vi "MultiplexerSerialInterfaceHost.vi"() -> ()   [LabVIEW 2016]
uses:
  <vilib>/FPGAPlugInAG/USB-7856R OEM/niLvFpga_Open_USB-7856R OEM.vi
  <vilib>/rvi/interface/common/dynamic/niFpgaDynamicAddResources.vi
  <vilib>/Utility/error.llb/Error Cluster From Error Code.vi
  <vilib>/rvi/errors/niLvFpgaAdjustHostInterfaceError.vi
  <vilib>/FPGAPlugInAG/Dynamic/niLvFpga_Close_Dynamic.vi
  <vilib>/rvi/interface/nirviOpenFPGA/nirviOpenFPGA.xnode
  FPGA Bitfiles/qnmController797_usbRIO_MultiplexerSPIFPGA.lvbitx
  <vilib>/rvi/interface/nirviReadWriteControl/nirviReadWriteControl.xnode
  <vilib>/rvi/interface/nirviCloseFPGA/nirviCloseFPGA.xnode
  NiFpgaLv.dll
  <vilib>/rvi/interface/Simulation/niFpgaSimulationCallBeginRW.vi
panel:
  in  "Buffer":T1={"Update Multiplexer"=FALSE, "Channel #"=0, "Dimension"=32, "Selection"=0, "Clock delay"=50} {"Selection" items=["AO0 (X)", "AO1 (Y)", "AO2 (Z)", "AO3 (DRIVE)", "AO4 (BIAS)", "AO5 (STICK-SLIP X - DC Motor)", "AO6 (STICK-SLIP Y)", "AO7 (STICK-SLIP Z )", "AI0 (Deflection)", "AI1 (Horizontal)", "AI2 (Sum)", "AI3", "AI4", "AI5", "AI6", "AI7"]; "Channel #" max=32}
  in  "Output Enable":bool
  in  "VGA":T2={"Update"=FALSE, "Dimension"=32, "Selection"=0, "Clock delay"=50, "Gain (dB)"=0} {"Gain (dB)" max=40; "Selection" items=["AO0 (X)", "AO1 (Y)", "AO2 (Z)", "AO3 (DRIVE)", "AO4 (BIAS)", "AO5 (STICK-SLIP X - DC Motor)", "AO6 (STICK-SLIP Y)", "AO7 (STICK-SLIP Z )", "AI0 (Deflection)", "AI1 (Horizontal)", "AI2 (Sum)", "AI3", "AI4", "AI5", "AI6", "AI7"]}
  in  "Multiplexer":T1={"Update Multiplexer"=FALSE, "Channel #"=0, "Dimension"=32, "Selection"=0, "Clock delay"=50} {"Selection" items=["AO0 (X)", "AO1 (Y)", "AO2 (Z)", "AO3 (DRIVE)", "AO4 (BIAS)", "AO5 (STICK-SLIP X - DC Motor)", "AO6 (STICK-SLIP Y)", "AO7 (STICK-SLIP Z )", "AI0 (Deflection)", "AI1 (Horizontal)", "AI2 (Sum)", "AI3", "AI4", "AI5", "AI6", "AI7"]; "Channel #" max=32}
  in  "Frequency":u16(ring) items=["AO0 (X)", "AO1 (Y)", "AO2 (Z)", "AO3 (DRIVE)", "AO4 (BIAS)", "AO5 (STICK-SLIP X - DC Motor)", "AO6 (STICK-SLIP Y)", "AO7 (STICK-SLIP Z )", "AI0 (Deflection)", "AI1 (Horizontal)", "AI2 (Sum)", "AI3", "AI4", "AI5", "AI6", "AI7"]
  in  "Clock delay 2":u32=50
  in  "Dimension 2":u8=32
  in  "Line #":u8 max=32
  in  "Update Quad Multiplier":bool
  # "Buffer"
  # "VGA"
  # "HMC960LP4E"
  # "DAC8554"
  # "Quad Multiplier"
  # "Multiplexer"
  # "HV5122"
  # "DAC8803"
  # "Select the element"
  # "Select the element"
  # "Select the element"
  # "Select the element"
  # "MICROCHIP"
  # "TEXAS INSTRUMENTS"
  # "Serial to Parallel Converter"
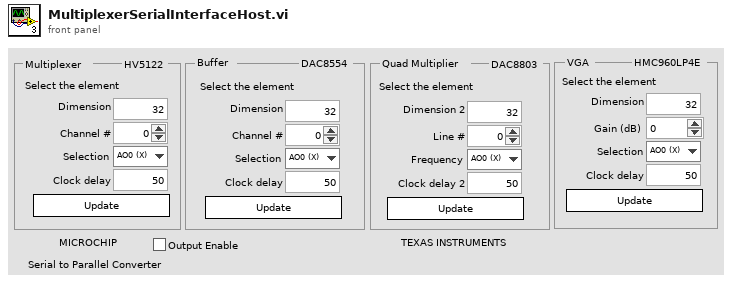
[diagram p1: front panel]
types:
  T1 = cluster{"Update Multiplexer":bool, "Channel #":u8, "Dimension":u8, "Selection":u16, "Clock delay":u32}
  T2 = cluster{"Update":bool, "Dimension":u8, "Selection":u16, "Clock delay":u32, "Gain (dB)":u32}
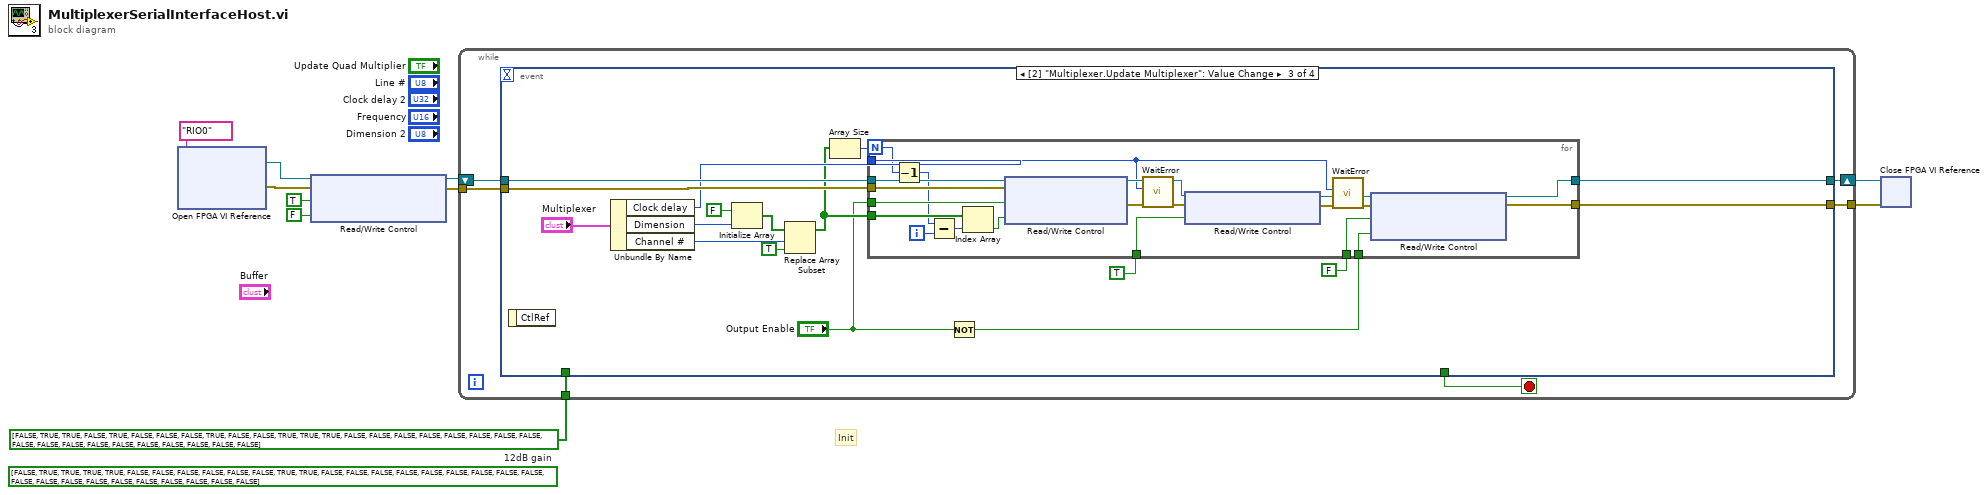
[diagram p0: block diagram]
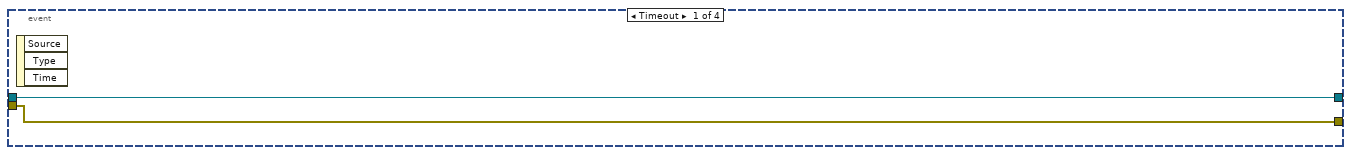
[diagram p2: hidden frame]
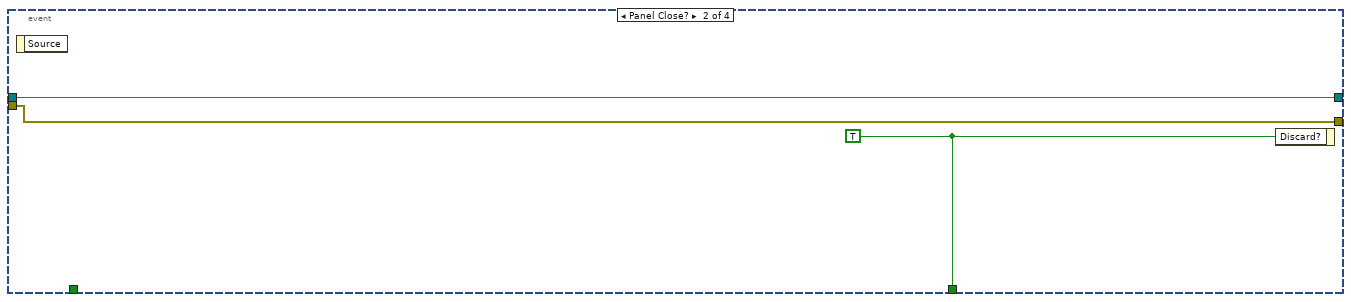
[diagram p3: hidden frame]
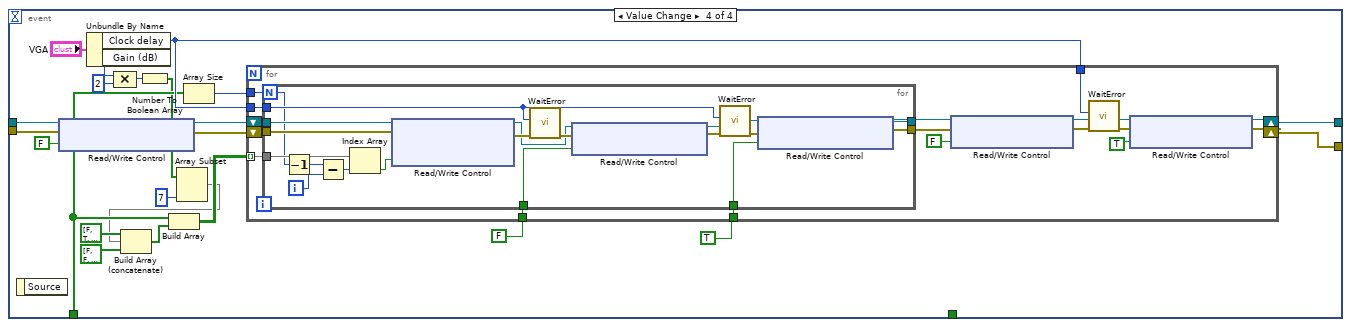
[diagram p4: hidden frame]
diagram:
  (unwired) bool[] [FALSE, TRUE, TRUE, TRUE, TRUE, FALSE, FALSE, FALSE, FALSE, FALSE, FALSE, TRUE, TRUE, FALSE, FALSE, FALSE, FALSE, FALSE, FALSE, FALSE, FALSE, FALSE, FALSE, FALSE, FALSE, FALSE, FALSE, FALSE, FALSE, FALSE, FALSE, FALSE]  # 12dB gain
  # "Init"
  n1 = xnode "Open FPGA VI Reference"("resource name"=tag "RIO0") -> ("FPGA VI Reference Out"=w8:refnum<k20>, "error out"=w5:errorcluster)  [unwired: 1 in]
  n2 = xnode "Read/Write Control"("FPGA VI Reference In"=w8, "error in"=w5, "dio.p.multiplexerOE"=TRUE ("dio.p.multiplexerclock"), "dio.p.multiplexerclock"=FALSE) -> ("FPGA VI Reference Out"=w7:refnum<k20>, "error out"=w6:errorcluster)
  n3 = while {
    tunnel: w6 -> [w14]
    shift-right: [w13] -> w4
    shift-left: w7 -> [w16]
    tunnel: [w12] -> w3
    tunnel: bool[] [FALSE, TRUE, TRUE, FALSE, TRUE, FALSE, FALSE, FALSE, TRUE, FALSE, FALSE, TRUE, TRUE, TRUE, FALSE, FALSE, FALSE, FALSE, FALSE, FALSE, FALSE, FALSE, FALSE, FALSE, FALSE, FALSE, FALSE, FALSE, FALSE, FALSE, FALSE, FALSE] ("output array") -> [w11]
    stop <- w15 stop-if-true
    n4 = event shown="[2] \"Multiplexer.Update Multiplexer\": Value Change" {
      selector: _ -> [_ _ _ _]
      dyn-events: _ -> [_ _ _ _]
      timeout: _ -> [_ _ _ _]
      tunnel: w16 -> [w18 w20 w37 w78]
      tunnel: [_ w21 _ _] -> w15
      tunnel: w14 -> [w17 w19 w36 w74]
      tunnel: [w18 w20 w34 w73] -> w13
      tunnel: [w17 w19 w25 w72] -> w12
      tunnel: w11 -> [_ _ _ w69]
      event Timeout {
        n5 = event-data() -> ()  [unwired: 1 in, 3 out]
      }
      event Panel Close? {
        w21 = TRUE ("Discard?")
        n6 = event-data() -> ()  [unwired: 1 in, 1 out]
        n7 = event-data("Discard?"=w21) -> ()  [unwired: 1 in, 1 out]
      }
      event "Multiplexer.Update Multiplexer": Value Change {
        n8 = event-data() -> ()  [unwired: 1 in, 1 out]
        n9 = Unbundle By Name("Multiplexer") -> ("Clock delay"=w27:u32, "Dimension"=w29:u8, "Channel #"=w28:u8)
        n10 = Initialize Array(FALSE, w29) -> (w31:bool[])
        n11 = Replace Array Subset(array=w31, new element=TRUE ("new element/subarray"), index=w28) -> (w26:bool[])
        n12 = Array Size(array=w26) -> (size(s)=w35:i32)
        n13 = Not(x="Output Enable") -> (.not. x?=w22:bool)
        n14 = for {
          N: w35 -> [w46]
          tunnel: w27 -> [w53]
          tunnel: w37 -> [w52]
          tunnel: w26 -> [w47]
          tunnel: "Output Enable" -> [w51]
          tunnel: w22 -> [w48]
          tunnel: TRUE ("dio.p.multiplexerclock") -> [w50]
          tunnel: w36 -> [w49]
          tunnel: [w43] -> w34
          tunnel: FALSE ("dio.p.multiplexerclock") -> [w42]
          tunnel: [w41] -> w25
          i -> [w45]
          n15 = Decrement(x=w46) -> (x-1=w39:i32)
          n16 = Subtract(x=w39, y=w45) -> (x-y=w44:i32)
          n17 = Index Array(array=w47, index=w44) -> (element=w40:bool)
          n18 = xnode "Read/Write Control"("FPGA VI Reference In"=w52, "error in"=w49, "dio.p.multiplexerOE"=w51, "dio.i.dataIn"=w40) -> ("FPGA VI Reference Out"=w54:refnum<k20>, "error out"=w59:errorcluster)
          n19 = call "WaitError.vi"("error in (no error)"=w59, "milliseconds to wait"=w53) -> ("error out"=w58:errorcluster)  [unwired: 9 in]
          n20 = xnode "Read/Write Control"("FPGA VI Reference In"=w54, "error in"=w58, "dio.p.multiplexerclock"=w50) -> ("FPGA VI Reference Out"=w55:refnum<k20>, "error out"=w57:errorcluster)
          n21 = call "WaitError.vi"("error in (no error)"=w57, "milliseconds to wait"=w53) -> ("error out"=w56:errorcluster)  [unwired: 9 in]
          n22 = xnode "Read/Write Control"("FPGA VI Reference In"=w55, "error in"=w56, "dio.p.multiplexerclock"=w42, "dio.p.multiplexerOE"=w48) -> ("FPGA VI Reference Out"=w43:refnum<k20>, "error out"=w41:errorcluster)
        }
      }
      event "VGA.Update": Value Change {
        n23 = event-data() -> ()  [unwired: 1 in, 1 out]
        n24 = xnode "Read/Write Control"("FPGA VI Reference In"=w78, "error in"=w74, "dio.p.multiplexerclock"=FALSE) -> ("FPGA VI Reference Out"=w77:refnum<k20>, "error out"=w75:errorcluster)
        n25 = Unbundle By Name("VGA") -> ("Clock delay"=w71:u32, "Gain (dB)"=w66:u32)
        n26 = Compound Arithmetic op=MULTIPLY(w66, u32 2 ("value")) -> (w65:u32)
        n27 = Number To Boolean Array(number=w65) -> (Boolean array=w63:bool[])
        n28 = Array Subset(array=w63, length=7) -> (w62:bool[])  [unwired: 1 in]
        n29 = Build Array (concatenate)(bool[] [FALSE, TRUE, TRUE, TRUE, TRUE, FALSE, FALSE, FALSE], w62, bool[] [FALSE, FALSE, FALSE, FALSE, FALSE, FALSE, FALSE, FALSE, FALSE]) -> (w68:bool[])
        n30 = Build Array(w69, w68) -> (w70:bool[][])
        n31 = Array Size(array=w69) -> (size(s)=w82:i32)
        n32 = for {
          tunnel: w82 -> [w99]
          tunnel: FALSE ("dio.p.multiplexerclock") -> [w98]
          tunnel: w71 -> [w97]
          tunnel: TRUE ("dio.p.multiplexerclock") -> [w96]
          tunnel: w70 -> [w93] mode=indexing
          shift-right: [w85] -> w73
          shift-left: w77 -> [w95]
          shift-right: [w84] -> w72
          shift-left: w75 -> [w94]
          tunnel: w71 -> [w83]
          n33 = for {
            N: w99 -> [w107]
            tunnel: w97 -> [w112]
            tunnel: w95 -> [w111]
            tunnel: w93 -> [w108]
            tunnel: w98 -> [w110]
            tunnel: w94 -> [w109]
            tunnel: [w104] -> w86
            tunnel: w96 -> [w103]
            tunnel: [w102] -> w87
            i -> [w106]
            n34 = Decrement(x=w107) -> (x-1=w100:i32)
            n35 = Subtract(x=w100, y=w106) -> (x-y=w105:i32)
            n36 = Index Array(array=w108, index=w105) -> (element=w101:bool)
            n37 = xnode "Read/Write Control"("FPGA VI Reference In"=w111, "error in"=w109, "dio.i.dataIn"=w101) -> ("FPGA VI Reference Out"=w113:refnum<k20>, "error out"=w118:errorcluster)  [unwired: 1 in]
            n38 = call "WaitError.vi"("error in (no error)"=w118, "milliseconds to wait"=w112) -> ("error out"=w117:errorcluster)  [unwired: 9 in]
            n39 = xnode "Read/Write Control"("FPGA VI Reference In"=w113, "error in"=w117, "dio.p.multiplexerclock"=w110) -> ("FPGA VI Reference Out"=w114:refnum<k20>, "error out"=w116:errorcluster)
            n40 = call "WaitError.vi"("error in (no error)"=w116, "milliseconds to wait"=w112) -> ("error out"=w115:errorcluster)  [unwired: 9 in]
            n41 = xnode "Read/Write Control"("FPGA VI Reference In"=w114, "error in"=w115, "dio.p.multiplexerclock"=w103) -> ("FPGA VI Reference Out"=w104:refnum<k20>, "error out"=w102:errorcluster)
          }
          n42 = xnode "Read/Write Control"("FPGA VI Reference In"=w86, "error in"=w87, "dio.p.multiplexerOE"=FALSE) -> ("FPGA VI Reference Out"=w89:refnum<k20>, "error out"=w90:errorcluster)
          n43 = call "WaitError.vi"("error in (no error)"=w90, "milliseconds to wait"=w83) -> ("error out"=w88:errorcluster)  [unwired: 9 in]
          n44 = xnode "Read/Write Control"("FPGA VI Reference In"=w89, "error in"=w88, "dio.p.multiplexerOE"=TRUE ("dio.i.dataIn")) -> ("FPGA VI Reference Out"=w85:refnum<k20>, "error out"=w84:errorcluster)
        }
      }
    }
  }
  n45 = xnode "Close FPGA VI Reference"("FPGA VI Reference In"=w4, "error in"=w3) -> ()  [unwired: 1 out]
